vi "Auto_Routine_LeaveRobotStartingZone.vi"(8 "error in (no error)":errorcluster) -> (0 "error out":errorcluster)   [LabVIEW 2023]
doc: "Leaves the community\n\ninput:\n--ErrorIn--\n\noutput:\n--ErrorOut--"
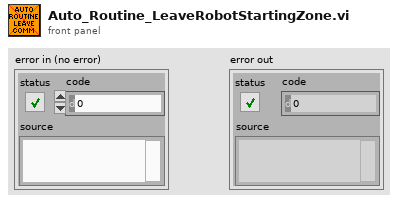
[diagram p1: front panel]
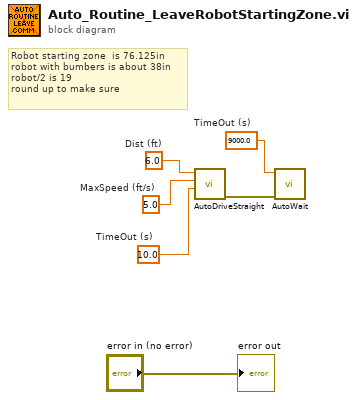
[diagram p0: block diagram]
diagram:
  w1 = 9000.0  # TimeOut (s)
  w3 = 10.0  # TimeOut (s)
  w4 = 6.0  # Dist (ft)
  w5 = 5.0  # MaxSpeed (ft/s)
  # "Robot starting zone  is 76.125in \nrobot with bumbers is about 38in\nrobot/2 is 19\nround up to make sure"
  n1 = call "AutoDriveStraight.vi"("TimeOut (s)"=w3, "MaxSpeed (ft/s)"=w5, "Dist (ft)"=w4) -> ("error out"=w2:errorcluster)  [unwired: 8 in]
  n2 = call "AutoWait.vi"("error in (no error)"=w2, "TimeOut (s)"=w1) -> ()  [unwired: 9 in, 1 out]
  "error out" <- "error in (no error)"
